vi "GetTerms3.vi"(0 "XRef":T10, 1 "State In":T9={"Input Type"=variant(dbl 0.0), "Selection"=0, "Element Names"=[], "Type Strings"=[], "Element Types"=[]}) -> (14 "Terms":T1)   [LabVIEW 2015, in "Construct-Tagged-Union.xnode"]
doc: "This ability VI is used to describe your terminals to LabVIEW. Terms is an array of clusters describing the XNode's terminals.\n ID: A unique string identifying the terminal.\n Name: The name of the terminal visible to the user. Remember to localize it.\n Type: The data type of the terminal (as a Variant). The data put in the variant will be used as the default for the input terminal if it's left unwired.\n Bounds: A rectangle defining the bounds of the terminal relative to the bounds of the XNode. The bounds must be within the bounds of the XNode, and for whiskers to draw properly, they must be flush with at least one side of the XNode.\n Input?: Indicates whether or not this terminals is an input.\n Required?: Indicates whether the user must wire this terminal for the XNode to not be broken. Ignored on outputs.\n Recommended?: Indicates whether the terminal is recommended.\n Hidden?: Indicates whether the terminal is hidden. When a terminal is hidden, it cannot be wired to via user interaction or scripting. However, if it is already wired to when the hidden flag is changed to true, it will remain wired.\n Adaptive?: Indicates that the term should change to match the type of its source if it is wired.\n Direction?: Indicates what direction the wire stub should point. Choose auto to let LV decide based on the terms bounds being on the nodes edge.\n \n The IDs are used by LabVIEW to keep track of your terminals. When you respecify your terminals, LabVIEW can tell whther terminals are new, deleted, or moved by the unique IDs. The order is irrelevant. If you move a terminal, then any wire connected to it will move with it.\n \n If you want to update your terminals, you should return the UpdateTerms reply in one of your ability VIs.\n\nDefault behavior: None.\n\nThis ability does not provide UI and OS messages are not handled."
uses:
  Construct-Tagged-Union.xnode
  <vilib>/XNodeSupport/XNodeXNodeRef.ctl
  State.ctl
  <vilib>/XNodeSupport/XNodeTerm3Array.ctl
  <vilib>/XNodeSupport/XNodeTerm3.ctl
  <vilib>/XNodeSupport/XNodeString.ctl
  <vilib>/XNodeSupport/XNodeVariant.ctl
  <vilib>/XNodeSupport/XNodeRect32.ctl
  <vilib>/XNodeSupport/XNodeInt.ctl
  <vilib>/XNodeSupport/XNodeBool.ctl
  <vilib>/XNodeSupport/XNodeTermDirection.ctl
  <vilib>/XNodeSupport/NI_XNodeSupport.lvlib
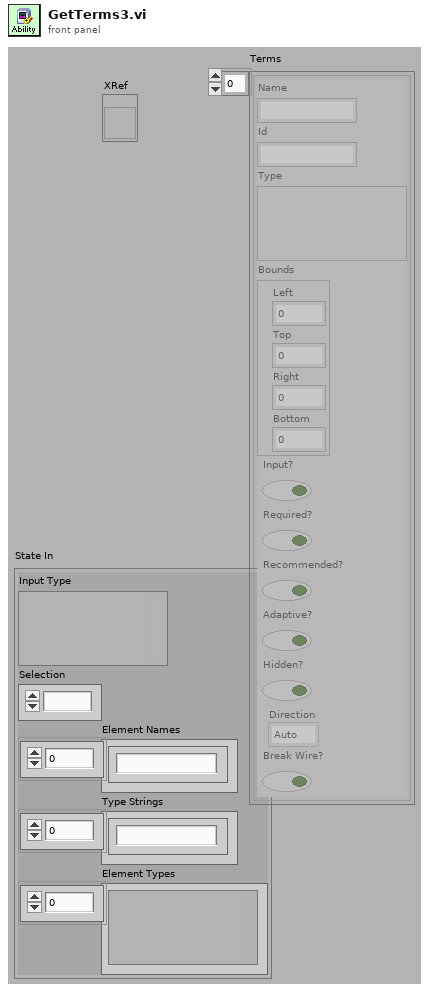
[diagram p1: front panel]
types:
  T1 = typedef "NI_XNodeSupport.lvlib/XNodeTerm3Array.ctl" = T2[]
  T2 = typedef "NI_XNodeSupport.lvlib/XNodeTerm3.ctl" = cluster{"Name":T3, "Id":T3, "Type":T4, "Bounds":T5, "Input?":T7, "Required?":T7, "Recommended?":T7, "Adaptive?":T7, "Hidden?":T7, "Direction":T8, "Break Wire?":T7}
  T3 = typedef "NI_XNodeSupport.lvlib/XNodeString.ctl" = string
  T4 = typedef "NI_XNodeSupport.lvlib/XNodeVariant.ctl" = variant
  T5 = typedef "NI_XNodeSupport.lvlib/XNodeRect32.ctl" = cluster{"Left":T6, "Top":T6, "Right":T6, "Bottom":T6}
  T6 = typedef "NI_XNodeSupport.lvlib/XNodeInt.ctl" = i32
  T7 = typedef "NI_XNodeSupport.lvlib/XNodeBool.ctl" = bool
  T8 = typedef "NI_XNodeSupport.lvlib/XNodeTermDirection.ctl" = enum32{"Auto", "Up", "Down", "Left", "Right", "Center"}
  T9 = typedef "Construct-Tagged-Union.xnode/State.ctl" = cluster{"Input Type":variant, "Selection":i32, "Element Names":string[], "Type Strings":string[], "Element Types":variant[]}
  T10 = typedef "NI_XNodeSupport.lvlib/XNodeXNodeRef.ctl" = refnum<vi>
  T11 = cluster{"left":i16, "top":i16, "right":i16, "bottom":i16}
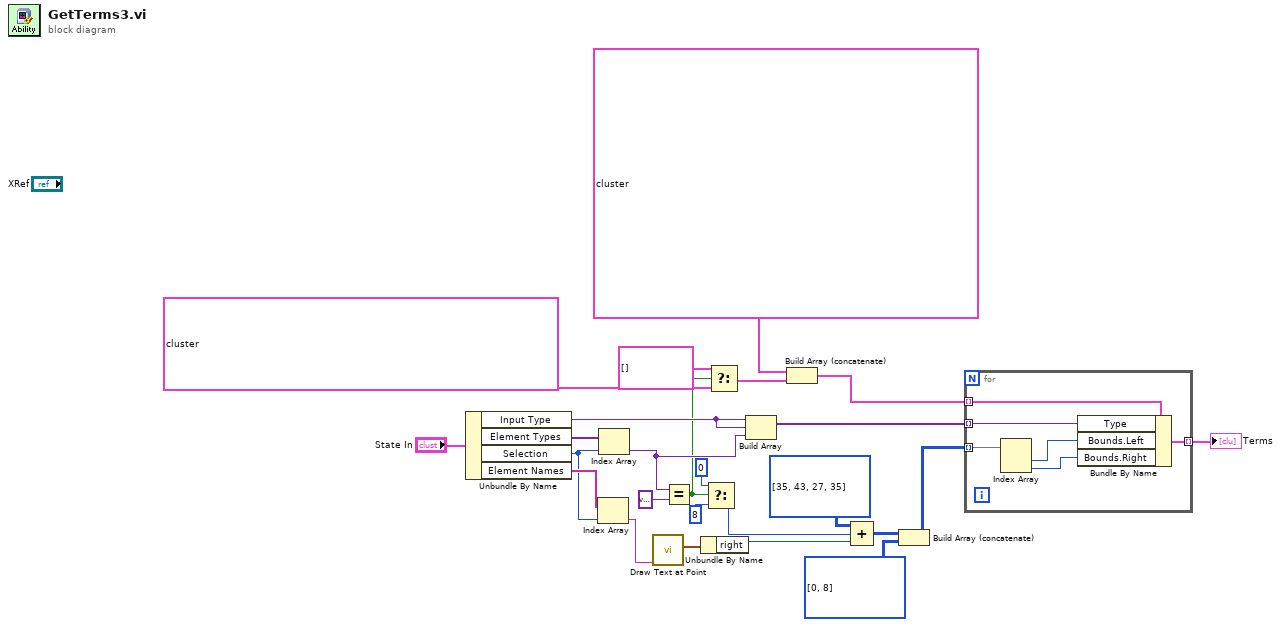
[diagram p0: block diagram]
diagram:
  n1 = Unbundle By Name("State In") -> ("Input Type"=w23:variant, "Element Types"=w19:variant[], "Selection"=w17:i32, "Element Names"=w18:string[])
  n2 = Index Array(array=w18, index=w17) -> (element=w16:string)
  n3 = Index Array(array=w19, index=w17) -> (element=w21:variant)
  n4 = call <vilib>:"Draw Text at Point.vi"("text"=w16) -> ("text rect"=w15:T11)  [unwired: 9 in, 1 out]
  n5 = Equal?(x=w21, y=variant) -> (x = y?=w6:bool)
  n6 = Unbundle By Name(w15) -> ("right"=w12:i16)
  n7 = Select(t=i16 0 ("right"), s=w6, f=i16 8 ("right")) -> (s? t:f=w11:i16)
  n8 = Select(t=T2[] [], s=w6, f=T2[] [{"Name"="in", "Id"="in", "Type"=variant, "Bounds"={"Left"=0, "Top"=5, "Right"=8, "Bottom"=13}, "Input?"=TRUE, "Required?"=TRUE, "Recommended?"=TRUE, "Adaptive?"=FALSE, "Hidden?"=FALSE, "Direction"=enum."Auto", "Break Wire?"=FALSE}]) -> (s? t:f=w3:T2[])
  n9 = Build Array(w23, w23, w21) -> (w25:variant[])
  n10 = Build Array (concatenate)(T2[] [{"Name"="Tagged Union out", "Id"="tout", "Type"=variant, "Bounds"={"Left"=86, "Top"=5, "Right"=98, "Bottom"=13}, "Input?"=FALSE, "Required?"=FALSE, "Recommended?"=TRUE, "Adaptive?"=FALSE, "Hidden?"=FALSE, "Direction"=enum."Right", "Break Wire?"=FALSE}, {"Name"="Type", "Id"="type", "Type"=variant, "Bounds"={"Left"=0, "Top"=0, "Right"=8, "Bottom"=8}, "Input?"=TRUE, "Required?"=TRUE, "Recommended?"=TRUE, "Adaptive?"=FALSE, "Hidden?"=FALSE, "Direction"=enum."Auto", "Break Wire?"=FALSE}], w3) -> (w1:T2[])
  n11 = Compound Arithmetic op=unknown(i16[][] [[35, 43], [27, 35]], w11, w12) -> (w9:i16[][])
  n12 = Build Array (concatenate)(w9, i16[][] [[0, 8]]) -> (w8:i16[][])
  n13 = for {
    tunnel: w1 -> [w31] mode=indexing
    tunnel: w25 -> [w29] mode=indexing
    tunnel: [w30] -> w22 mode=indexing
    tunnel: w8 -> [w28] mode=indexing
    n14 = Index Array(array=w28) -> (element #1=w27:i16, element #2=w26:i16)  [unwired: 2 in]
    n15 = Bundle By Name(cluster=w31, "Type"=w29, "Bounds.Left"=w27, "Bounds.Right"=w26) -> (w30:T2)
  }
  "Terms" <- w22
